vi "EventClient_GetEvent.vi"(8 "error in (no error)":errorcluster, 9 "timeout in ms (-1)":i32=-1, 11 "reference":T1) -> (0 "error out":errorcluster, 1 "Data":variant, 2 "Name":string, 3 "reference out":T1, 5 "timed out?":bool)   [LabVIEW 2018]
uses:
  EventClient_ObjectReference.ctl
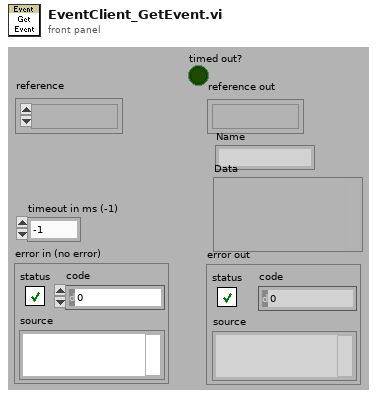
[diagram p1: front panel]
types:
  T1 = typedef "EventClient_ObjectReference.ctl" = refnum<k1>
  T2 = cluster{"Client":refnum<queue>, "Sub Events":string[], "PrvData":variant, "MyName":string}
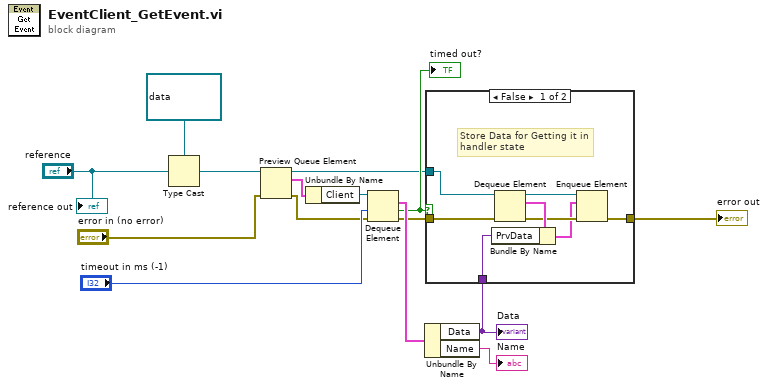
[diagram p0: block diagram]
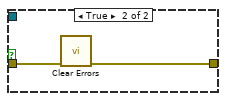
[diagram p2: hidden frame]
diagram:
  n1 = Type Cast(type=refnum<queue> refnum ("queue out"), x="reference") -> (*(type *) &x=w14:refnum<queue>)
  n2 = Preview Queue Element(queue=w14, error in (no error)="error in (no error)") -> (queue out=w3:refnum<queue>, element=w13:T2, error out=w9:errorcluster)  [unwired: 2 out]
  n3 = Unbundle By Name(w13) -> ("Client"=w11:refnum<queue>)
  n4 = Dequeue Element(queue=w11, timeout in ms (-1)="timeout in ms (-1)", error in (no error)=w9) -> (element=w8:cluster{"Name":string, "Data":variant}, timed out?=w6:bool, error out=w5:errorcluster)  [unwired: 1 out]
  "timed out?" <- w6
  n5 = Unbundle By Name(w8) -> ("Data"=w2:variant, "Name"=→"Name":string)
  "Data" <- w2
  n6 = case shown="False" w6 {
    tunnel: w5 -> [w23 w25]
    tunnel: [w17 w24] -> w4
    tunnel: w3 -> [w22 _]
    tunnel: w2 -> [w20 _]
    frame False {
      # "Store Data for Getting it in handler state"
      n7 = Dequeue Element(queue=w22, error in (no error)=w23) -> (queue out=w19:refnum<queue>, element=w21:T2, error out=w18:errorcluster)  [unwired: 2 out]
      n8 = Bundle By Name(cluster=w21, "PrvData"=w20) -> (w16:T2)
      n9 = Enqueue Element(queue=w19, element=w16, error in (no error)=w18) -> (error out=w17:errorcluster)  [unwired: 3 out]
    }
    frame True {
      n10 = call <vilib>:"Clear Errors.vi"("error in (no error)"=w25) -> ("error out"=w24:errorcluster)  [unwired: 1 in, 5 out]
    }
  }
  "error out" <- w4
  "reference out" <- "reference"
